vi "com spex.vi"() -> ()   [LabVIEW 2009]
uses:
  <vilib>/Instr/_visa.llb/VISA Configure Serial Port (Instr).vi
panel:
  in  "write par":string
  in  "milliseconds to wait":u32=50
  out "Numeric":i32
  out "concatenated string":string
  in  "com/par":bool
  in  "write com":string
  in  "Boolean":bool
  out "error out":errorcluster
  in  "stop":bool
  out "return count":u32
  out "read buffer":string
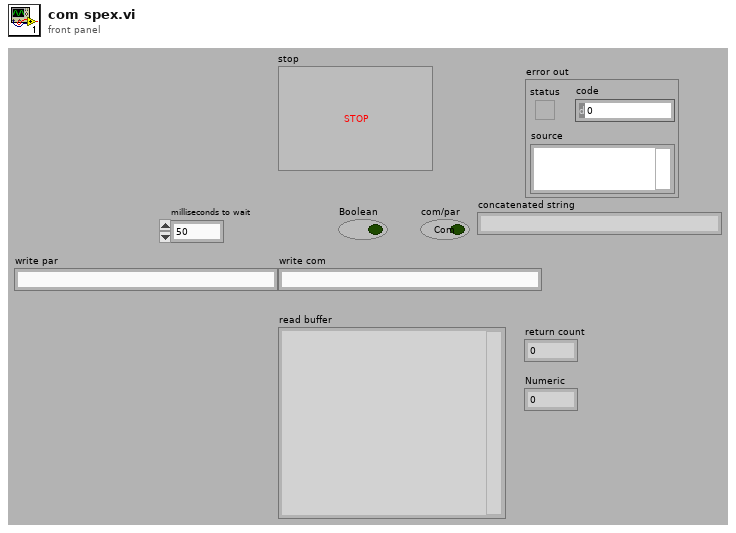
[diagram p1: front panel]
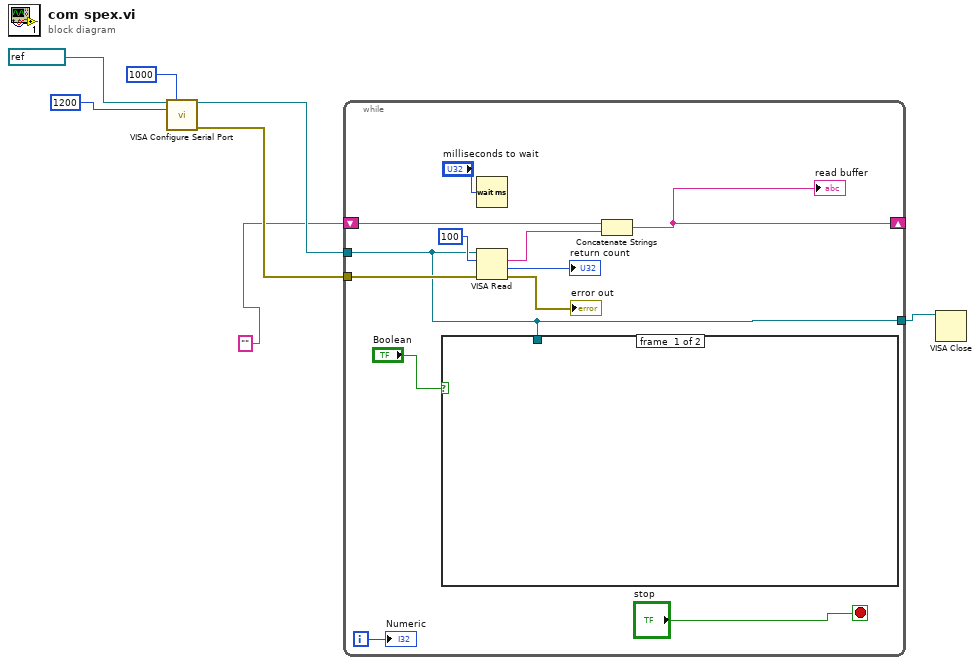
[diagram p0: block diagram]
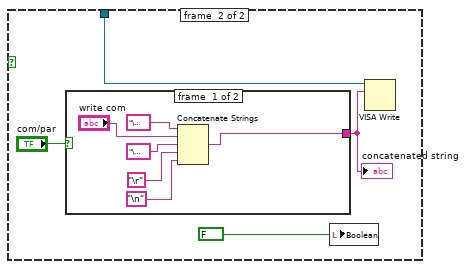
[diagram p2: hidden frame]
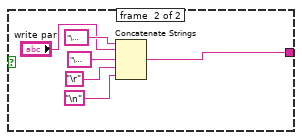
[diagram p3: hidden frame]
diagram:
  n1 = call-poly "VISA Configure Serial Port"("VISA resource name"=refnum<visa-resource-name> "COM1", "timeout (10sec)"=u32 1000, "baud rate (9600)"=u32 1200) -> ("VISA resource name out"=w5:refnum<visa-resource-name>, "error out"=w4:errorcluster)  [unwired: 11 in]
  n2 = while {
    tunnel: w5 -> [w8]
    tunnel: w4 -> [w19]
    shift-right: [w13] -> _
    shift-left: "" -> [w12]
    tunnel: [w8] -> w1
    i -> [w9]
    stop <- "stop" stop-if-true
    n3 = case shown="True" "Boolean" {
      tunnel: w8 -> [_ w22]
      frame #0 {
      }
      frame #1 {
        n4 = case shown="False" "com/par" {
          tunnel: [w25 w31] -> w20
          frame #0 {
            n5 = Concatenate Strings("\u0018" ("string"), "write com", "\u0003" ("string"), "\r", "\n") -> (w25:string)
          }
          frame #1 {
            n6 = Concatenate Strings("\u0002" ("string"), "write par", "\u0003" ("string"), "\r", "\n") -> (w31:string)
          }
        }
        "concatenated string" <- w20
        n7 = local write "Boolean"(FALSE ("Boolean")) -> ()
        n8 = VISA Write(VISA resource name=w22, write buffer=w20) -> ()  [unwired: 1 in, 3 out]
      }
    }
    n9 = Wait (ms)(milliseconds to wait="milliseconds to wait") -> ()  [unwired: 1 out]
    n10 = VISA Read(VISA resource name=w8, byte count=u32 100, error in (no error)=w19) -> (read buffer=w11:string, return count=→"return count":u32, error out=→"error out":errorcluster)  [unwired: 1 out]
    n11 = Concatenate Strings(w12, w11) -> (w13:string)
    "read buffer" <- w13
    "Numeric" <- w9
  }
  n12 = VISA Close(VISA resource name=w1) -> ()  [unwired: 1 in, 1 out]
